vi "asg8100序列编辑.vi"() -> ()   [LabVIEW 2018]
uses:
  <vilib>/Utility/miscctls.llb/LVRowAndColumnTypeDef.ctl
panel:
  in  "json缓存":string
  out "图表转数据":i32[][](array[numeric])
  in  "停止":bool
  out "最大行数":i32
  in  "路径":path
  in  "多列列表框":i32[](listbox)
  out "单元格位置":T1
  in  "清除":bool
  in  "添加行":bool
  in  "保存文件":bool
  in  "加载文加":bool
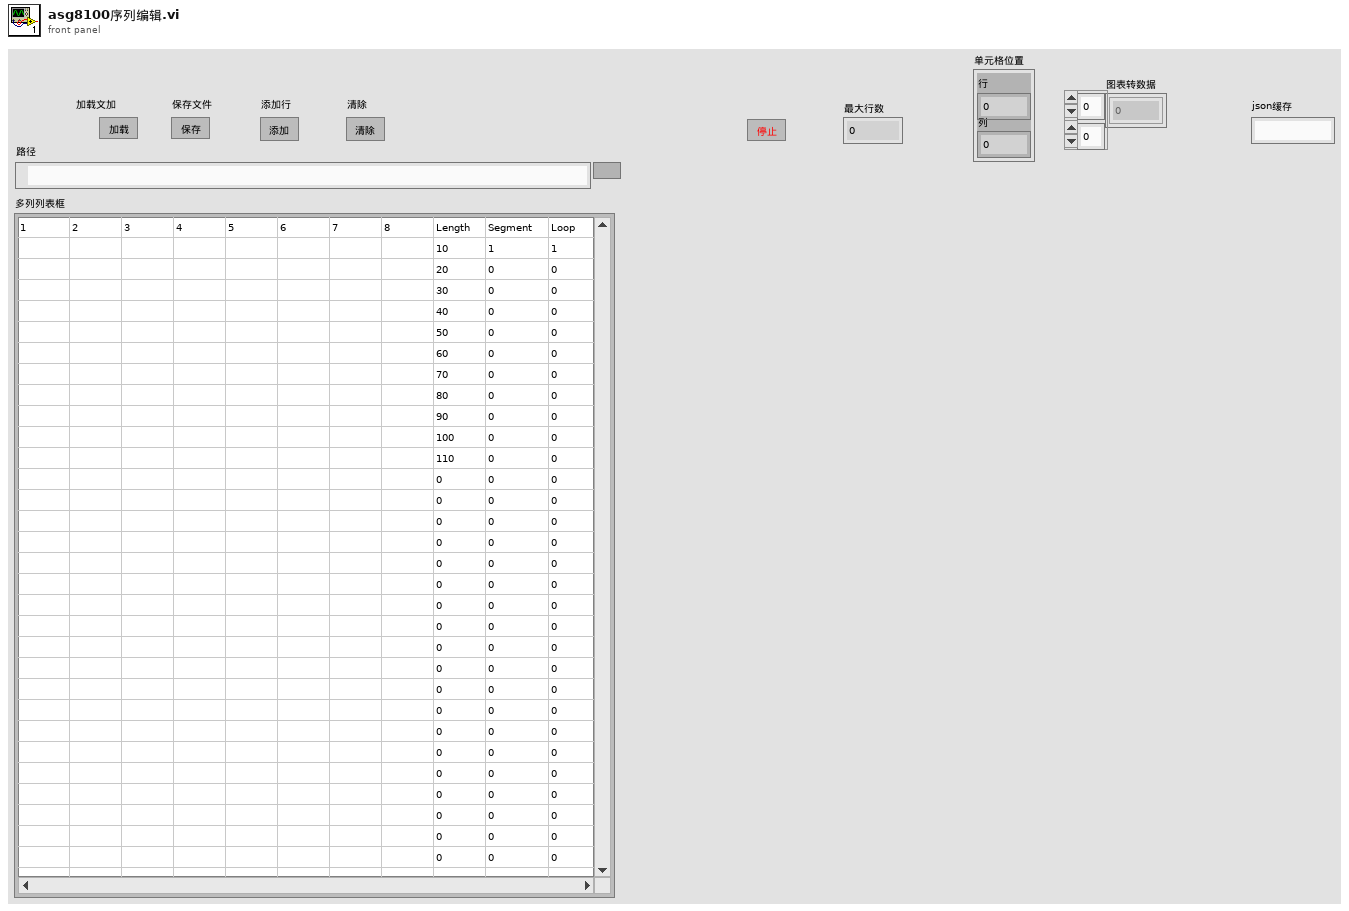
[diagram p1: front panel]
types:
  T1 = typedef "LVRowAndColumnTypeDef.ctl" = cluster{"Row":i32, "Column":i32}
  T2 = typedef "LVPoint32TypeDef.ctl" = cluster{"Horizontal":i32, "Vertical":i32}
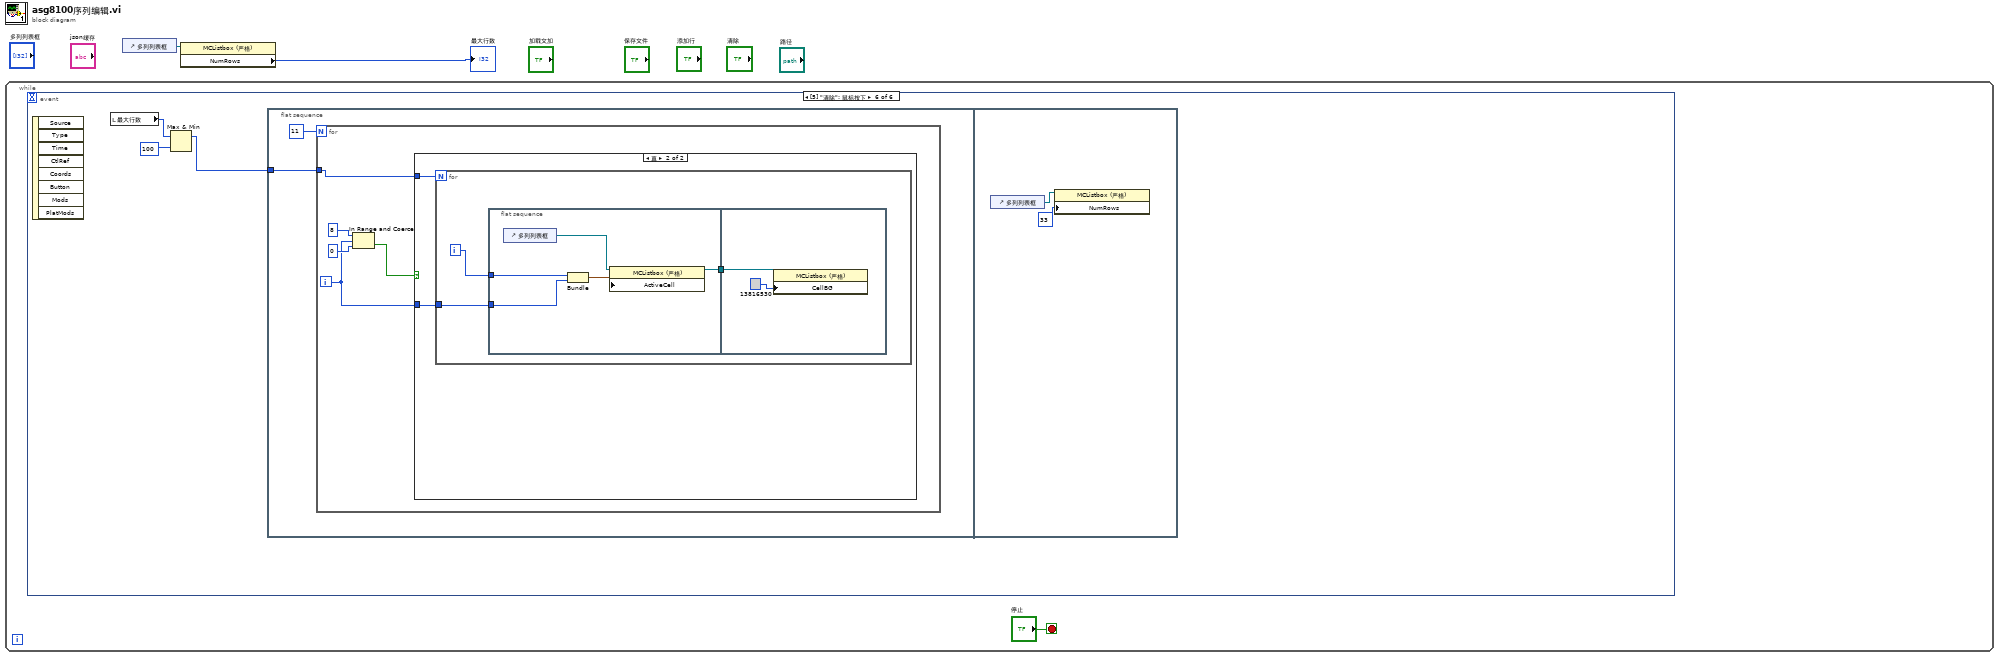
[diagram p0: block diagram]
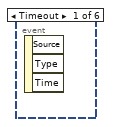
[diagram p2: hidden frame]
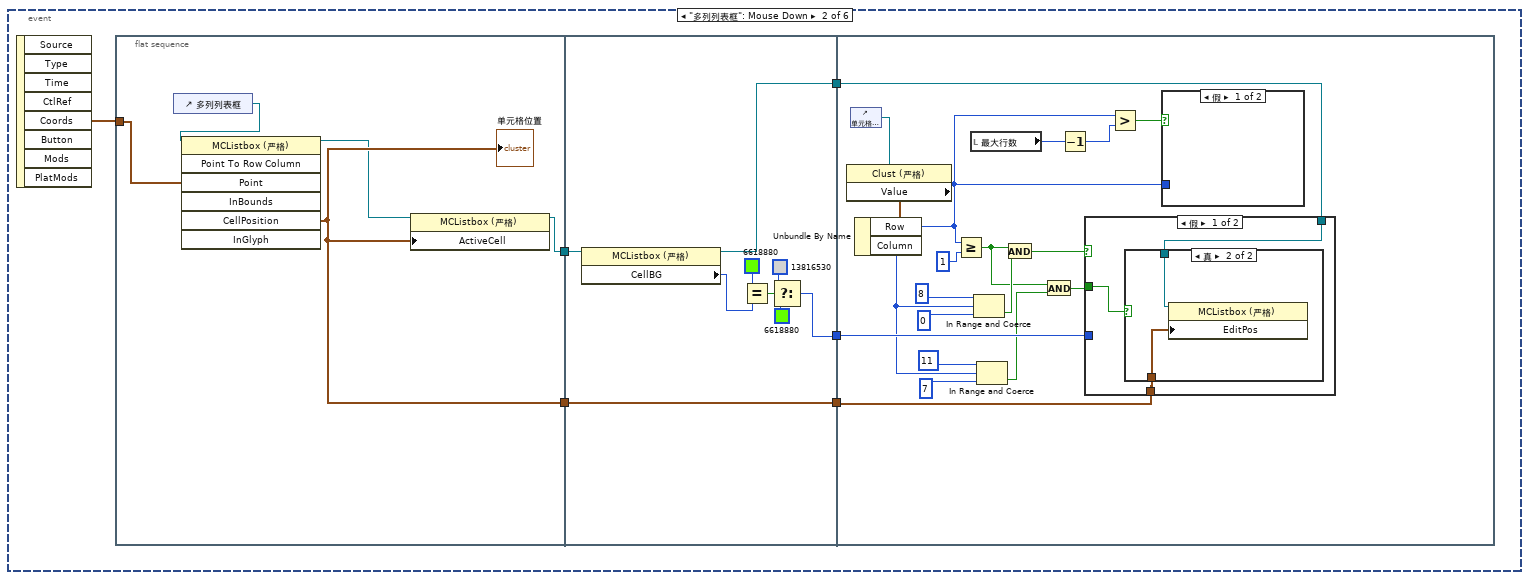
[diagram p3: hidden frame]
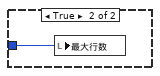
[diagram p4: hidden frame]
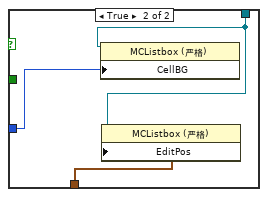
[diagram p6: hidden frame]
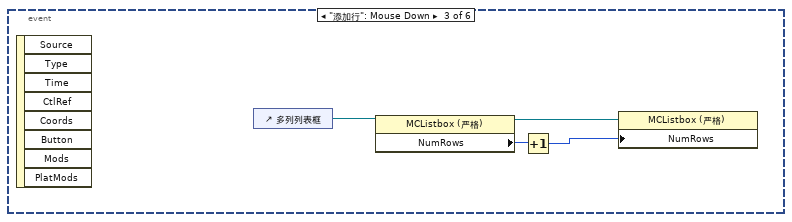
[diagram p7: hidden frame]
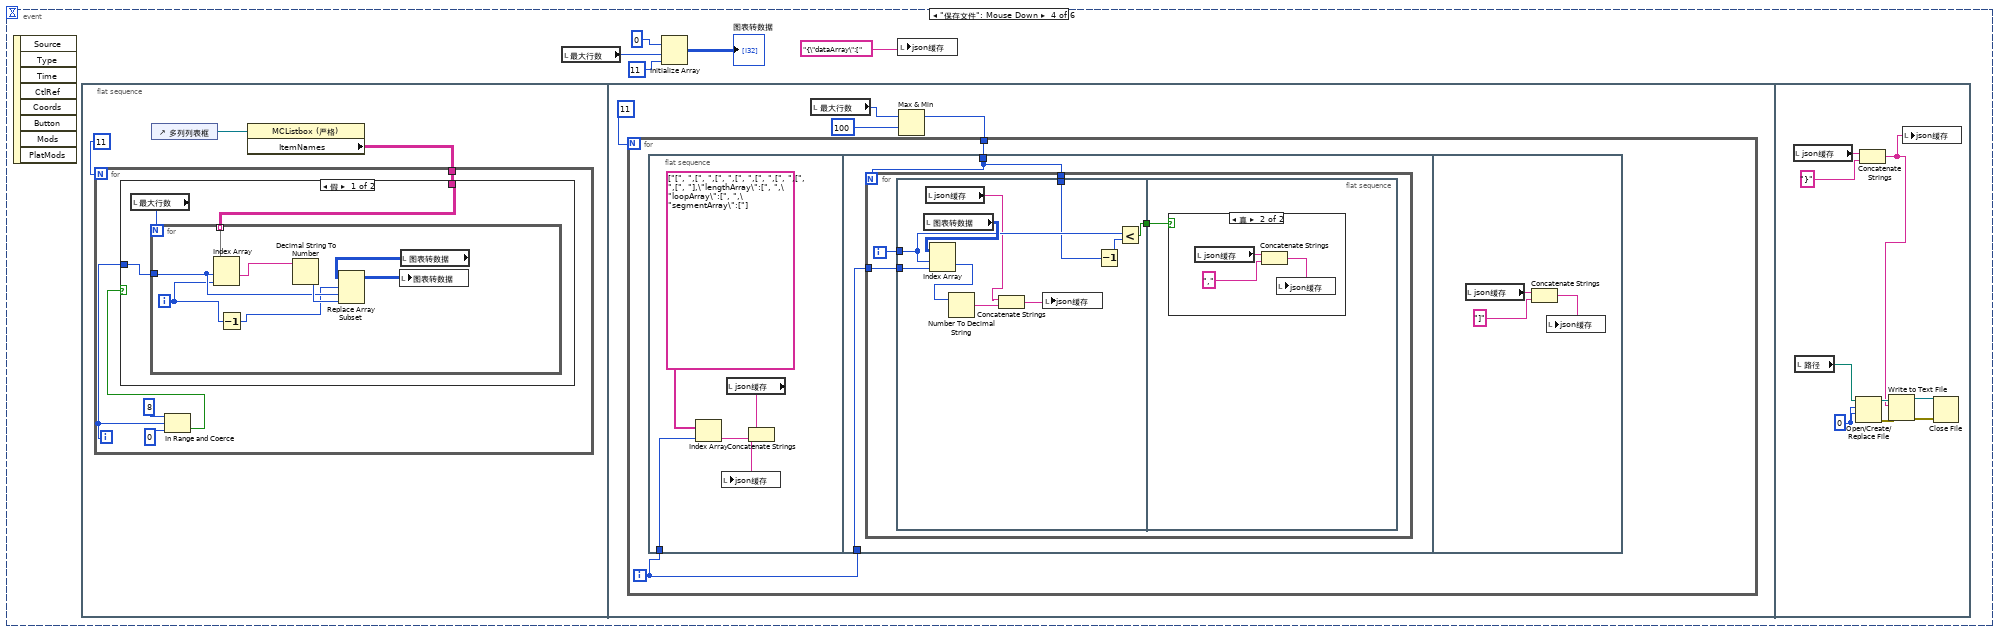
[diagram p8: hidden frame]
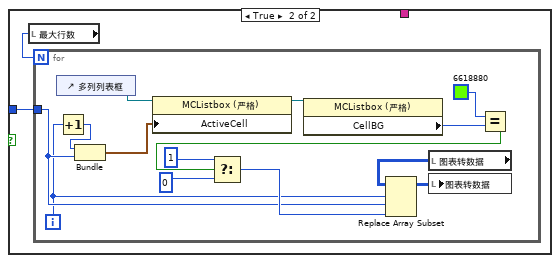
[diagram p9: hidden frame]
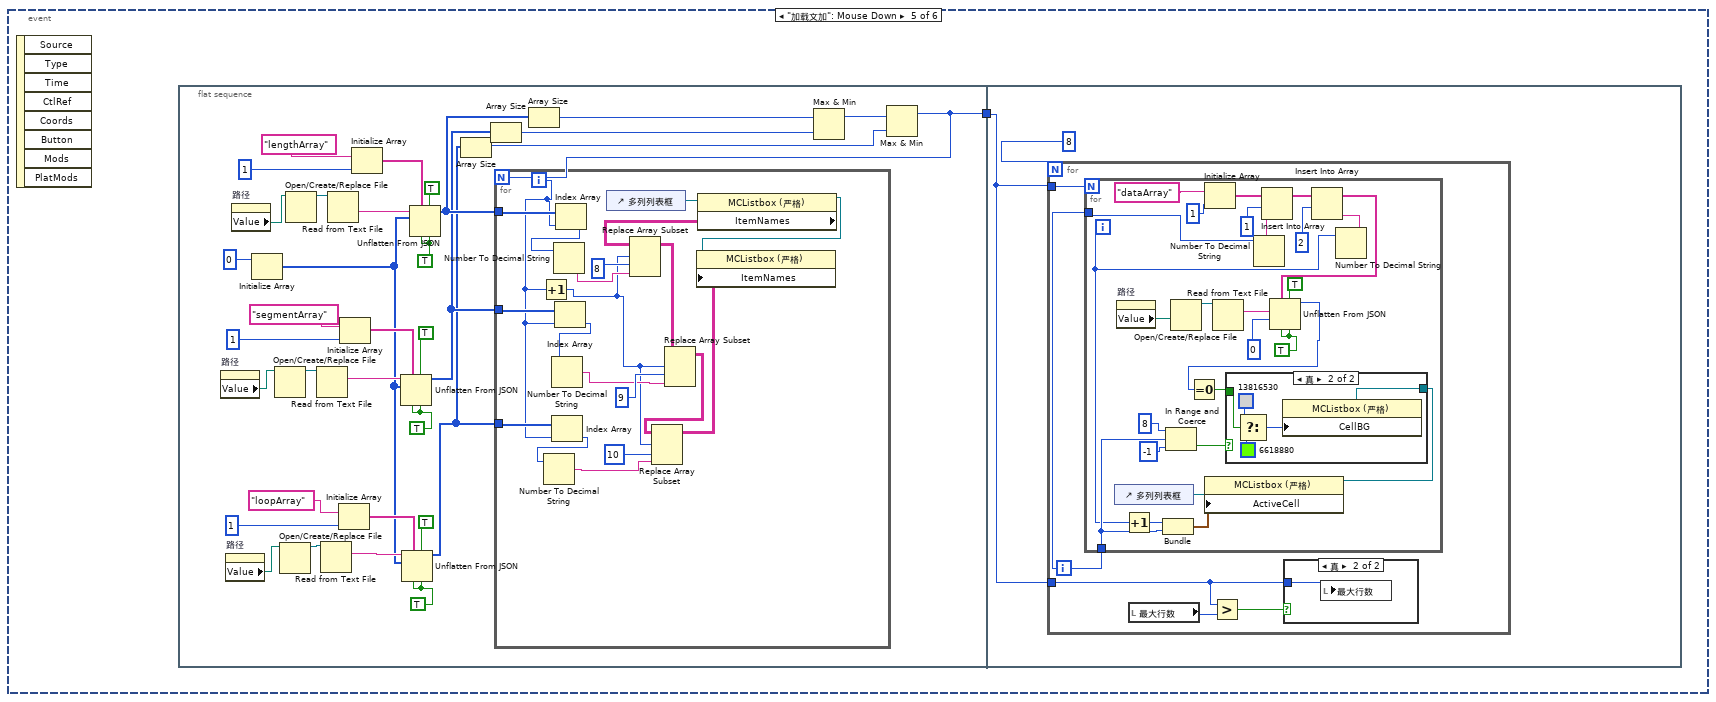
[diagram p11: hidden frame]
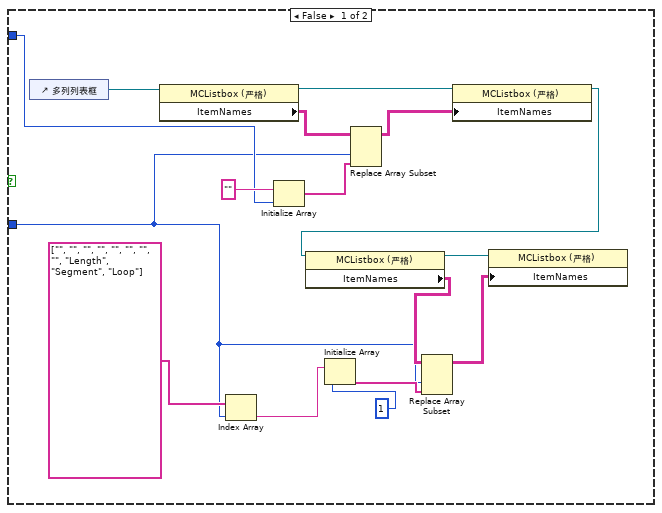
[diagram p14: hidden frame]
diagram:
  n1 = while {
    stop <- "停止" stop-if-true
    n2 = event shown="[5] \"清除\": 鼠标按下" {
      selector: _ -> [_ _ _ _ _ _]
      dyn-events: _ -> [_ _ _ _ _ _]
      timeout: _ -> [_ _ _ _ _ _]
      event Timeout {
        n3 = event-data() -> ()  [unwired: 1 in, 3 out]
      }
      event "多列列表框": Mouse Down {
        n4 = event-data() -> ("Coords"=w6:T2)  [unwired: 1 in, 7 out]
        n5 = flat-sequence {
          tunnel: [w10] -> w9
          tunnel: w6 -> [w13]
          tunnel: [w14] -> w5
          tunnel: w9 -> [w19]
          tunnel: [w16] -> w8
          tunnel: [w18] -> w7
          tunnel: w5 -> [w15]
          tunnel: [w15] -> w4
          tunnel: w8 -> [w43]
          tunnel: w7 -> [w42]
          tunnel: w4 -> [w30]
          frame #0 {
            n6 = control-ref of="多列列表框"() -> (w12:refnum<vi>)
            n7 = invoke class="MCListbox (严格)" method="Point To Row Column"(reference=w12, "Point"=w13) -> (reference out=w11:refnum<vi>, "CellPosition"=w14:T1)  [unwired: 5 in, 5 out]
            "单元格位置" <- w14
            n8 = property class="MCListbox (严格)"(reference=w11, "ActiveCell"=w14) -> (reference out=w10:refnum<vi>)  [unwired: 1 in, 1 out]
          }
          frame #1 {
            n9 = property class="MCListbox (严格)"(reference=w19) -> (reference out=w16:refnum<vi>, "CellBG"=w22:u32)  [unwired: 1 in, 1 out]
            n10 = Equal?(x=u32 6618880, y=w22) -> (x = y?=w23:bool)
            n11 = Select(t=u32 13816530, s=w23, f=u32 6618880) -> (s? t:f=w18:u32)
          }
          frame #2 {
            n12 = control-ref of="单元格位置"() -> (w41:refnum<vi>)
            n13 = property class="Clust (严格)"(reference=w41) -> ("Value"=w40:T1)  [unwired: 1 in, 2 out]
            n14 = Unbundle By Name(w40) -> ("Row"=w29:i32, "Column"=w33:i32)
            n15 = Greater Or Equal?(x=w29, y=1) -> (x >= y?=w31:bool)
            n16 = local read "最大行数"() -> (w26:i32)
            n17 = In Range and Coerce(upper limit=8, x=w33, lower limit=0) -> (In Range?=w36:bool)  [unwired: 1 out]
            n18 = In Range and Coerce(upper limit=11, x=w33, lower limit=7) -> (In Range?=w32:bool)  [unwired: 1 out]
            n19 = And(x=w31, y=w36) -> (x .and. y?=w37:bool)
            n20 = And(x=w31, y=w32) -> (x .and. y?=w27:bool)
            n21 = Decrement(x=w26) -> (x-1=w25:i32)
            n22 = case shown="假" w37 {
              tunnel: w43 -> [w46 w51]
              tunnel: w42 -> [_ w52]
              tunnel: w27 -> [w47 _]
              tunnel: w30 -> [w45 w50]
              frame False {
                n23 = case shown="真" w47 {
                  tunnel: w46 -> [_ w49]
                  tunnel: w45 -> [_ w48]
                  frame False {
                  }
                  frame True {
                    n24 = property class="MCListbox (严格)"(reference=w49, "EditPos"=w48) -> ()  [unwired: 1 in, 2 out]
                  }
                }
              }
              frame True {
                n25 = property class="MCListbox (严格)"(reference=w51, "CellBG"=w52) -> ()  [unwired: 1 in, 2 out]
                n26 = property class="MCListbox (严格)"(reference=w51, "EditPos"=w50) -> ()  [unwired: 1 in, 2 out]
              }
            }
            n27 = Greater?(x=w29, y=w25) -> (0:w28:bool)
            n28 = case shown="假" w28 {
              tunnel: w29 -> [_ w44]
              frame False {
              }
              frame True {
                n29 = local write "最大行数"(w44) -> ()
              }
            }
          }
        }
      }
      event "添加行": Mouse Down {
        n30 = event-data() -> ()  [unwired: 1 in, 8 out]
        n31 = control-ref of="多列列表框"() -> (w56:refnum<vi>)
        n32 = property class="MCListbox (严格)"(reference=w56) -> (reference out=w53:refnum<vi>, "NumRows"=w55:u32)  [unwired: 1 in, 1 out]
        n33 = Increment(x=w55) -> (x+1=w54:u32)
        n34 = property class="MCListbox (严格)"(reference=w53, "NumRows"=w54) -> ()  [unwired: 1 in, 2 out]
      }
      event "保存文件": Mouse Down {
        n35 = event-data() -> ()  [unwired: 1 in, 8 out]
        n36 = flat-sequence {
          frame #0 {
            n37 = control-ref of="多列列表框"() -> (w63:refnum<vi>)
            n38 = property class="MCListbox (严格)"(reference=w63) -> ("ItemNames"=w62:string[][])  [unwired: 1 in, 2 out]
            n39 = for {
              N: 11 -> [_]
              tunnel: w62 -> [w65]
              i -> [w66]
              n40 = In Range and Coerce(upper limit=8, x=w66, lower limit=0) -> (In Range?=w68:bool)  [unwired: 1 out]
              n41 = case shown="假" w68 {
                tunnel: w66 -> [w70 w81]
                tunnel: w65 -> [w72 _]
                frame False {
                  n42 = local read "最大行数"() -> (w71:i32)
                  n43 = for {
                    N: w71 -> [_]
                    tunnel: w72 -> [w77] mode=indexing
                    tunnel: w70 -> [w75]
                    i -> [w74]
                    n44 = Index Array(array=w77, index #1=w75, index #2=w74) -> (element #1=w76:string)  [unwired: 1 out]
                    n45 = Decrement(x=w74) -> (x-1=w73:i32)
                    n46 = Decimal String To Number(string=w76) -> (number=w79:i32)  [unwired: 2 in, 1 out]
                    n47 = local read "图表转数据"() -> (w80:i32[][])
                    n48 = Replace Array Subset(array=w80, new element=w79, index (row)=w73, index (col)=w75) -> (w78:i32[][])
                    n49 = local write "图表转数据"(w78) -> ()
                  }
                }
                frame True {
                  n50 = local read "最大行数"() -> (w82:i32)
                  n51 = for {
                    N: w82 -> [_]
                    tunnel: w81 -> [w85]
                    i -> [w84]
                    n52 = control-ref of="多列列表框"() -> (w96:refnum<vi>)
                    n53 = Increment(x=w84) -> (x+1=w83:i32)
                    n54 = Bundle(w83, w85) -> (w92:cluster{i32, i32})  [unwired: 1 in]
                    n55 = property class="MCListbox (严格)"(reference=w96, "ActiveCell"=w92) -> (reference out=w95:refnum<vi>)  [unwired: 1 in, 1 out]
                    n56 = property class="MCListbox (严格)"(reference=w95) -> ("CellBG"=w94:u32)  [unwired: 1 in, 2 out]
                    n57 = local read "图表转数据"() -> (w91:i32[][])
                    n58 = Equal?(x=u32 6618880, y=w94) -> (x = y?=w88:bool)
                    n59 = Select(t=1, s=w88, f=0) -> (s? t:f=w86:i32)
                    n60 = Replace Array Subset(array=w91, new element=w86, index (row)=w84, index (col)=w85) -> (w87:i32[][])
                    n61 = local write "图表转数据"(w87) -> ()
                  }
                }
              }
            }
          }
          frame #1 {
            n62 = local read "最大行数"() -> (w98:i32)
            n63 = Max & Min(x=w98, y=100) -> (max(x,y)=w99:i32)  [unwired: 1 out]
            n64 = for {
              N: 11 -> [_]
              tunnel: w99 -> [w102]
              i -> [w101]
              n65 = flat-sequence {
                tunnel: w101 -> [w103]
                tunnel: w102 -> [w108]
                tunnel: w101 -> [w109]
                frame #0 {
                  n66 = Index Array(array=string[] ["[", ",[", ",[", ",[", ",[", ",[", ",[", ",[", "],\"lengthArray\":[", ",\"loopArray\":[", ",\"segmentArray\":["], index=w103) -> (element=w107:string)
                  n67 = local read "json缓存"() -> (w106:string)
                  n68 = Concatenate Strings(w106, w107) -> (w105:string)
                  n69 = local write "json缓存"(w105) -> ()
                }
                frame #1 {
                  n70 = for {
                    N: w108 -> [_]
                    tunnel: w109 -> [w113]
                    tunnel: w108 -> [w110]
                    i -> [w112]
                    n71 = flat-sequence {
                      tunnel: w113 -> [w122]
                      tunnel: w112 -> [w119]
                      tunnel: [w117] -> w111
                      tunnel: w110 -> [w114]
                      tunnel: w111 -> [w124]
                      frame #0 {
                        n72 = local read "图表转数据"() -> (w123:i32[][])
                        n73 = local read "json缓存"() -> (w116:string)
                        n74 = Index Array(array=w123, index (row)=w119, index (col)=w122) -> (element=w121:i32)
                        n75 = Number To Decimal String ("数值至十进制数字符串转换")(number=w121) -> (decimal integer string=w120:string)  [unwired: 1 in]
                        n76 = Concatenate Strings(w116, w120) -> (w115:string)
                        n77 = local write "json缓存"(w115) -> ()
                        n78 = Decrement(x=w114) -> (x-1=w118:i32)
                        n79 = Less?(x=w119, y=w118) -> (x < y?=w117:bool)
                      }
                      frame #1 {
                        n80 = case shown="真" w124 {
                          frame False {
                          }
                          frame True {
                            n81 = local read "json缓存"() -> (w127:string)
                            n82 = Concatenate Strings(w127, ",") -> (w125:string)
                            n83 = local write "json缓存"(w125) -> ()
                          }
                        }
                      }
                    }
                  }
                }
                frame #2 {
                  n84 = local read "json缓存"() -> (w128:string)
                  n85 = Concatenate Strings(w128, "]") -> (w130:string)
                  n86 = local write "json缓存"(w130) -> ()
                }
              }
            }
          }
          frame #2 {
            w133 = 0
            n87 = local read "json缓存"() -> (w139:string)
            n88 = local read "路径"() -> (w132:path)
            n89 = Open/Create/Replace File(file path (use dialog)=w132, operation (0:open)=w133, access (0:read/write)=w133) -> (refnum out=w134:refnum<file>, error out=w135:errorcluster)  [unwired: 3 in, 1 out]
            n90 = Concatenate Strings(w139, "}") -> (w131:string)
            n91 = Write to Text File(file (use dialog)=w134, text=w131, error in=w135) -> (refnum out=w136:refnum<file>, error out=w137:errorcluster)  [unwired: 1 in, 1 out]
            n92 = local write "json缓存"(w131) -> ()
            n93 = Close File(refnum=w136, error in=w137) -> ()  [unwired: 2 out]
          }
        }
        n94 = local read "最大行数"() -> (w59:i32)
        n95 = Initialize Array(0, w59, 11) -> (→"图表转数据":i32[][])
        n96 = local write "json缓存"("{\"dataArray\":[") -> ()
      }
      event "加载文加": Mouse Down {
        n97 = event-data() -> ()  [unwired: 1 in, 8 out]
        n98 = flat-sequence {
          tunnel: [w143] -> w140
          tunnel: w140 -> [w195]
          frame #0 {
            w161 = TRUE
            w166 = TRUE
            w173 = TRUE
            n99 = property on="路径" class="Path"() -> ("Value"=w168:path)  [unwired: 2 in, 2 out]
            n100 = property on="路径" class="Path"() -> ("Value"=w163:path)  [unwired: 2 in, 2 out]
            n101 = property on="路径" class="Path"() -> ("Value"=w171:path)  [unwired: 2 in, 2 out]
            n102 = Initialize Array(0) -> (w148:i32[])  [unwired: 1 in]
            n103 = Open/Create/Replace File(file path (use dialog)=w168) -> (refnum out=w167:refnum<file>)  [unwired: 5 in, 2 out]
            n104 = Open/Create/Replace File(file path (use dialog)=w163) -> (refnum out=w162:refnum<file>)  [unwired: 5 in, 2 out]
            n105 = Open/Create/Replace File(file path (use dialog)=w171) -> (refnum out=w172:refnum<file>)  [unwired: 5 in, 2 out]
            n106 = Read from Text File(file (use dialog)=w167) -> (text=w169:string)  [unwired: 3 in, 3 out]
            n107 = Read from Text File(file (use dialog)=w162) -> (text=w164:string)  [unwired: 3 in, 3 out]
            n108 = Read from Text File(file (use dialog)=w172) -> (text=w170:string)  [unwired: 3 in, 3 out]
            n109 = Initialize Array("loopArray", 1) -> (w153:string[])
            n110 = Initialize Array("segmentArray", 1) -> (w152:string[])
            n111 = Initialize Array("lengthArray", 1) -> (w151:string[])
            n112 = Unflatten From JSON(path=w152, enable LabVIEW extensions? (T)=TRUE, JSON string=w169, type and defaults=w148, default null elements? (F)=w166, strict validation? (F)=w166) -> (value=w142:i32[])  [unwired: 1 in, 1 out]
            n113 = Unflatten From JSON(path=w153, enable LabVIEW extensions? (T)=TRUE, JSON string=w164, type and defaults=w148, default null elements? (F)=w161, strict validation? (F)=w161) -> (value=w141:i32[])  [unwired: 1 in, 1 out]
            n114 = Unflatten From JSON(path=w151, enable LabVIEW extensions? (T)=TRUE, JSON string=w170, type and defaults=w148, default null elements? (F)=w173, strict validation? (F)=w173) -> (value=w144:i32[])  [unwired: 1 in, 1 out]
            n115 = Array Size(array=w141) -> (size(s)=w145:i32)
            n116 = Array Size(array=w142) -> (size(s)=w146:i32)
            n117 = Array Size(array=w144) -> (size(s)=w147:i32)
            n118 = Max & Min(x=w147, y=w146) -> (max(x,y)=w150:i32)  [unwired: 1 out]
            n119 = Max & Min(x=w150, y=w145) -> (max(x,y)=w143:i32)  [unwired: 1 out]
            n120 = for {
              N: w143 -> [_]
              tunnel: w144 -> [w194]
              tunnel: w142 -> [w187]
              tunnel: w141 -> [w185]
              i -> [w175]
              n121 = Increment(x=w175) -> (x+1=w176:i32)
              n122 = Index Array(array=w185, index=w175) -> (element=w183:i32)
              n123 = Number To Decimal String ("数值至十进制数字符串转换")(number=w183) -> (decimal integer string=w182:string)  [unwired: 1 in]
              n124 = Index Array(array=w187, index=w175) -> (element=w177:i32)
              n125 = Number To Decimal String ("数值至十进制数字符串转换")(number=w177) -> (decimal integer string=w178:string)  [unwired: 1 in]
              n126 = Index Array(array=w194, index=w175) -> (element=w193:i32)
              n127 = Number To Decimal String ("数值至十进制数字符串转换")(number=w193) -> (decimal integer string=w192:string)  [unwired: 1 in]
              n128 = control-ref of="多列列表框"() -> (w188:refnum<vi>)
              n129 = property class="MCListbox (严格)"(reference=w188) -> (reference out=w190:refnum<vi>, "ItemNames"=w189:string[][])  [unwired: 1 in, 1 out]
              n130 = Replace Array Subset(array=w189, new element=w192, index (row)=w176, index (col)=8) -> (w181:string[][])
              n131 = Replace Array Subset(array=w181, new element=w178, index (row)=w176, index (col)=9) -> (w180:string[][])
              n132 = Replace Array Subset(array=w180, new element=w182, index (row)=w176, index (col)=10) -> (w179:string[][])
              n133 = property class="MCListbox (严格)"(reference=w190, "ItemNames"=w179) -> ()  [unwired: 1 in, 2 out]
            }
          }
          frame #1 {
            n134 = for {
              N: 8 -> [_]
              tunnel: w195 -> [w201]
              tunnel: w195 -> [w199]
              i -> [w200]
              n135 = for {
                N: w201 -> [_]
                tunnel: w200 -> [w221]
                tunnel: w200 -> [w205]
                i -> [w203]
                w226 = TRUE
                n136 = control-ref of="多列列表框"() -> (w214:refnum<vi>)
                n137 = property on="路径" class="Path"() -> ("Value"=w228:path)  [unwired: 2 in, 2 out]
                n138 = Increment(x=w203) -> (x+1=w204:i32)
                n139 = Bundle(w204, w205) -> (w212:cluster{i32, i32})  [unwired: 1 in]
                n140 = In Range and Coerce(upper limit=8, x=w205, lower limit=-1) -> (In Range?=w209:bool)  [unwired: 1 out]
                n141 = Open/Create/Replace File(file path (use dialog)=w228) -> (refnum out=w229:refnum<file>)  [unwired: 5 in, 2 out]
                n142 = Initialize Array("dataArray", 1) -> (w223:string[])
                n143 = property class="MCListbox (严格)"(reference=w214, "ActiveCell"=w212) -> (reference out=w213:refnum<vi>)  [unwired: 1 in, 1 out]
                n144 = Read from Text File(file (use dialog)=w229) -> (text=w227:string)  [unwired: 3 in, 3 out]
                n145 = Number To Decimal String ("数值至十进制数字符串转换")(number=w221) -> (decimal integer string=w220:string)  [unwired: 1 in]
                n146 = Insert Into Array(array=w223, index=1, new element=w220) -> (w218:string[])
                n147 = Number To Decimal String ("数值至十进制数字符串转换")(number=w203) -> (decimal integer string=w219:string)  [unwired: 1 in]
                n148 = Insert Into Array(array=w218, index=2, new element=w219) -> (w215:string[])
                n149 = Unflatten From JSON(path=w215, enable LabVIEW extensions? (T)=TRUE, JSON string=w227, type and defaults=0, default null elements? (F)=w226, strict validation? (F)=w226) -> (value=w207:i32)  [unwired: 1 in, 1 out]
                n150 = Equal To 0?(x=w207) -> (x = 0?=w208:bool)
                n151 = case shown="真" w209 {
                  tunnel: w213 -> [_ w234]
                  tunnel: w208 -> [_ w230]
                  frame False {
                  }
                  frame True {
                    n152 = Select(t=u32 13816530, s=w230, f=u32 6618880) -> (s? t:f=w231:u32)
                    n153 = property class="MCListbox (严格)"(reference=w234, "CellBG"=w231) -> ()  [unwired: 1 in, 2 out]
                  }
                }
              }
              n154 = local read "最大行数"() -> (w198:i32)
              n155 = Greater?(x=w199, y=w198) -> (0:w197:bool)
              n156 = case shown="真" w197 {
                tunnel: w199 -> [_ w202]
                frame False {
                }
                frame True {
                  n157 = local write "最大行数"(w202) -> ()
                }
              }
            }
          }
        }
      }
      event "清除": Mouse Down {
        n158 = event-data() -> ()  [unwired: 1 in, 8 out]
        n159 = local read "最大行数"() -> (w237:i32)
        n160 = Max & Min(x=w237, y=100) -> (max(x,y)=w235:i32)  [unwired: 1 out]
        n161 = flat-sequence {
          tunnel: w235 -> [w238]
          frame #0 {
            n162 = for {
              N: 11 -> [_]
              tunnel: w238 -> [w240]
              i -> [w241]
              n163 = In Range and Coerce(upper limit=8, x=w241, lower limit=0) -> (In Range?=w242:bool)  [unwired: 1 out]
              n164 = case shown="真" w242 {
                tunnel: w241 -> [w245 w262]
                tunnel: w240 -> [w254 w261]
                frame False {
                  n165 = control-ref of="多列列表框"() -> (w258:refnum<vi>)
                  n166 = property class="MCListbox (严格)"(reference=w258) -> (reference out=w260:refnum<vi>, "ItemNames"=w257:string[][])  [unwired: 1 in, 1 out]
                  n167 = Index Array(array=string[] ["", "", "", "", "", "", "", "", "Length", "Segment", "Loop"], index=w245) -> (element=w248:string)
                  n168 = Initialize Array("", w254) -> (w255:string[])
                  n169 = Initialize Array(w248, 1) -> (w252:string[])
                  n170 = Replace Array Subset(array=w257, new element=w255, index (col)=w245) -> (w256:string[][])  [unwired: 1 in]
                  n171 = property class="MCListbox (严格)"(reference=w260, "ItemNames"=w256) -> (reference out=w253:refnum<vi>)  [unwired: 1 in, 1 out]
                  n172 = property class="MCListbox (严格)"(reference=w253) -> (reference out=w246:refnum<vi>, "ItemNames"=w251:string[][])  [unwired: 1 in, 1 out]
                  n173 = Replace Array Subset(array=w251, new element=w252, index (col)=w245) -> (w250:string[][])  [unwired: 1 in]
                  n174 = property class="MCListbox (严格)"(reference=w246, "ItemNames"=w250) -> ()  [unwired: 1 in, 2 out]
                }
                frame True {
                  n175 = for {
                    N: w261 -> [_]
                    tunnel: w262 -> [w264]
                    i -> [w263]
                    n176 = flat-sequence {
                      tunnel: [w269] -> w265
                      tunnel: w264 -> [w268]
                      tunnel: w263 -> [w267]
                      tunnel: w265 -> [w272]
                      frame #0 {
                        n177 = control-ref of="多列列表框"() -> (w266:refnum<vi>)
                        n178 = Bundle(w267, w268) -> (w270:cluster{i32, i32})  [unwired: 1 in]
                        n179 = property class="MCListbox (严格)"(reference=w266, "ActiveCell"=w270) -> (reference out=w269:refnum<vi>)  [unwired: 1 in, 1 out]
                      }
                      frame #1 {
                        n180 = property class="MCListbox (严格)"(reference=w272, "CellBG"=u32 13816530) -> ()  [unwired: 1 in, 2 out]
                      }
                    }
                  }
                }
              }
            }
          }
          frame #1 {
            n181 = control-ref of="多列列表框"() -> (w274:refnum<vi>)
            n182 = property class="MCListbox (严格)"(reference=w274, "NumRows"=33) -> ()  [unwired: 1 in, 2 out]
          }
        }
      }
    }
  }
  n183 = control-ref of="多列列表框"() -> (w2:refnum<vi>)
  n184 = property class="MCListbox (严格)"(reference=w2) -> ("NumRows"=→"最大行数":u32)  [unwired: 1 in, 2 out]
